vi "insert_data.vi"() -> ()   [LabVIEW 2019]
uses:
  <vilib>/addons/database/Connection.llb/DB Tools Open Connec (Path).vi
  <vilib>/addons/database/NI_Database_API.lvlib
panel:
  in  "temp":string
  in  "data":string
  in  "id":string
  in  "connection information":path
  in  "table":string
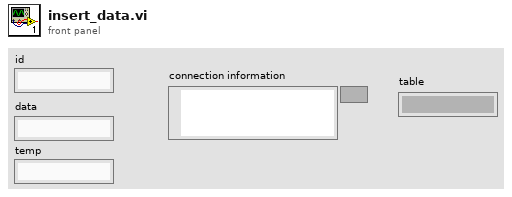
[diagram p1: front panel]
types:
  T1 = cluster{"id":string, "data":string, "temp":string}
  T2 = typedef "NI_Database_API.lvlib/Conn ObjectReference.ctl" = refnum<k1>
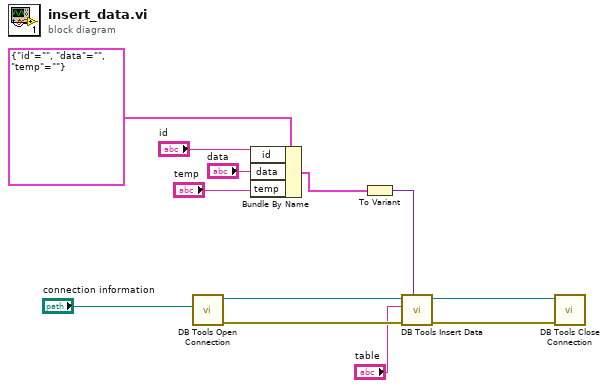
[diagram p0: block diagram]
diagram:
  n1 = call-poly <vilib>:"DB Tools Open Connection.vi"("connection information"="connection information") -> ("error out"=w9:errorcluster, "connection reference"=w10:T2)  [unwired: 7 in]
  n2 = Bundle By Name(cluster=T1 {"id"="", "data"="", "temp"=""}, "id"="id", "data"="data", "temp"="temp") -> (w6:T1)
  n3 = To Variant(anything=w6) -> (Variant=w8:variant)
  n4 = call <vilib>:"DB Tools Insert Data.vi"("data"=w8, "error in (no error)"=w9, "table"="table", "connection reference"=w10) -> ("error out"=w11:errorcluster, "connection reference out"=w12:T2)  [unwired: 6 in]
  n5 = call <vilib>:"DB Tools Close Connection.vi"("error in (no error)"=w11, "connection reference"=w12) -> ()  [unwired: 5 in, 1 out]
